vi "Edit CDMA Channel Setup.vi"(0 "VISA Resource Name":refnum<visa-resource-name>, 5 "Code Domain Power (0:IS-97)":enum16{"IS-97", "EQUAL", "SCALE", "NONE"}(ring), 7 "CDMA Setup":T1(array[cluster]) {"User Data" format="%.0b"; "Power" format="%.2f"}, 11 "error in (no error)":errorcluster {"code" format="%.0x"}) -> (4 "VISA Resource Name Out":refnum<visa-resource-name>, 15 "error out":errorcluster {"code" format="%.0x"})   [LabVIEW 2014, in "Agilent ESG Series.lvlib"]
doc: "This VI is used to configure the channel parameters.\nThe number of channel configurations sent to the instrument will equal the number of elements in the array.\n\nThis VI is valid only on instruments with the UND and UN5 options or on instrument E4438C with option 401."
uses:
  Agilent ESG Series.lvlib
panel:
  # "RANDOM\n\nUSER"
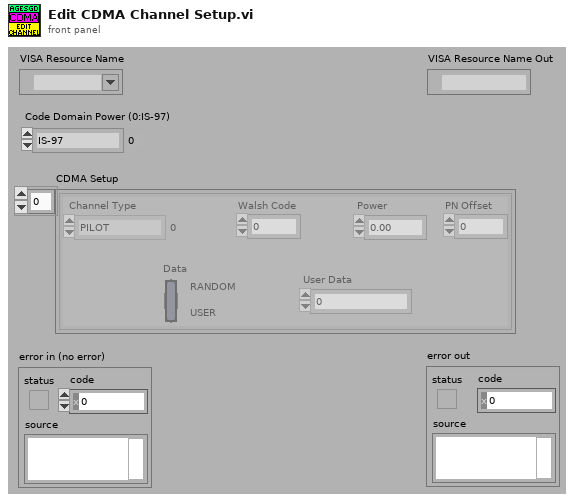
[diagram p1: front panel]
types:
  T1 = cluster{"Channel Type":enum16{"PILOT", "SYNC", "PAGING", "TRAFFIC"}, "Walsh Code":i32, "Power":dbl, "PN Offset":i32, "Data":bool, "User Data":i32}[]
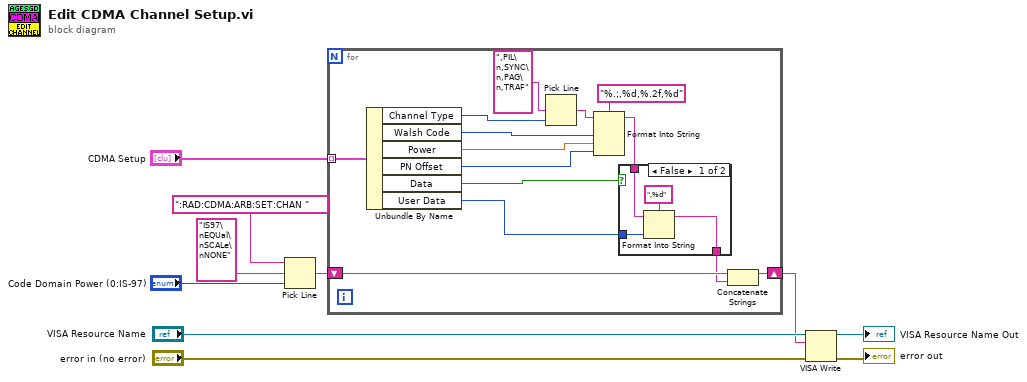
[diagram p0: block diagram]
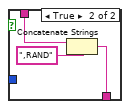
[diagram p2: hidden frame]
diagram:
  n1 = Pick Line(string ("")=":RAD:CDMA:ARB:SET:CHAN ", multi-line string="IS97\nEQUal\nSCALe\nNONE", line index="Code Domain Power (0:IS-97)") -> (output string=w3:string)
  n2 = for {
    tunnel: "CDMA Setup" -> [w16] mode=indexing
    shift-right: [w23] -> w4
    shift-left: w3 -> [w24]
    n3 = Unbundle By Name(w16) -> ("Channel Type"=w21:enum16{"PILOT", "SYNC", "PAGING", "TRAFFIC"}, "Walsh Code"=w15:i32, "Power"=w14:dbl, "PN Offset"=w13:i32, "Data"=w12:bool, "User Data"=w11:i32)
    n4 = Pick Line(multi-line string=",PIL\n,SYNC\n,PAG\n,TRAF", line index=w21) -> (output string=w20:string)  [unwired: 1 in]
    n5 = Format Into String(format string="%.;,%d,%.2f,%d", initial string=w20, w15, w14, w13) -> (resulting string=w18:string)  [unwired: 1 in, 1 out]
    n6 = case shown="False" w12 {
      tunnel: w18 -> [w28 w30]
      tunnel: w11 -> [w26 _]
      tunnel: [w25 w29] -> w17
      frame False {
        n7 = Format Into String(format string=",%d", initial string=w28, w26) -> (resulting string=w25:string)  [unwired: 1 in, 1 out]
      }
      frame True {
        n8 = Concatenate Strings(w30, ",RAND") -> (w29:string)
      }
    }
    n9 = Concatenate Strings(w24, w17) -> (w23:string)
  }
  n10 = VISA Write(VISA resource name="VISA Resource Name", write buffer=w4, error in (no error)="error in (no error)") -> (VISA resource name out=→"VISA Resource Name Out":refnum<visa-resource-name>, error out=→"error out":errorcluster)  [unwired: 1 out]
